vi "Main.vi"() -> ()   [LabVIEW 2021]
uses:
  Enum.ctl
  <vilib>/Instr/_visa.llb/VISA Configure Serial Port (Instr).vi
panel:
  in  "Zapisz Wykresy":bool
  in  "Wyczysc Wykresy":bool
  out "Temperatura Srednia Min [oC]":dbl
  out "PH10":cluster{"Output Value":dbl, dbl, dbl}(graph)
  out "p":cluster{"Output Value":dbl, dbl, dbl}(graph)
  out "RH":cluster{"Output Value":dbl, dbl, dbl}(graph)
  out "T":cluster{"Output Value":dbl, dbl, dbl}(graph)
  out "Iteracje Pomiarowe":i32
  out "Zapylenie Srednie Godz [ug/m3]":dbl
  out "Cisnienie Srednie Godz [hPa]":dbl
  out "Wilgotnosc Srednia Godz [%]":dbl
  out "Temperatura Srednia Godz [oC]":dbl
  out "Zapylenie Srednie Min [ug/m3]":dbl
  out "Cisnienie Srednie Min [hPa]":dbl
  out "Wilgotnosc Srednia Min [%]":dbl
  out "Zapylenie [ug/m3]":dbl
  in  "Potwierdz Haslo":bool
  in  "Haslo":string
  out "Cisnienie [hPa]":dbl
  out "Wilgotnosc [%]":dbl
  out "Temperatura [oC]":dbl
  out "Iteracje Programu":i32
  in  "Stop":bool
  in  "Arduino Port":refnum<visa-resource-name>
  # "Stacja Pogodowa"
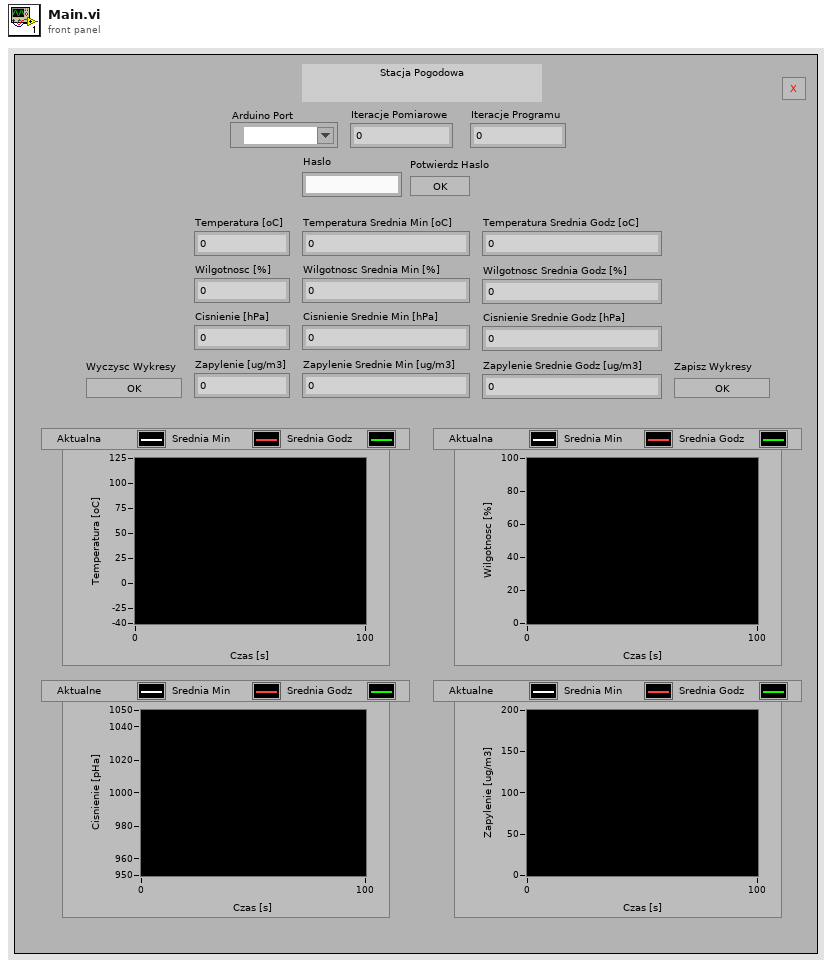
[diagram p1: front panel]
types:
  T1 = typedef "Enum.ctl" = enum16{"Init", "Password", "Measurement", "Save"}
  T2 = cluster{"Output Value":dbl, "Output Value":dbl, "Output Value":dbl, "Output Value":dbl}
  T3 = cluster{"Average 1":dbl, "Average 2":dbl, "Average 3":dbl, "Average 4":dbl}
  T4 = cluster{"Array 1":dbl[], "Array 2":dbl[], "Array 3":dbl[], "Array 4":dbl[]}
  T5 = cluster{"Output Value":dbl, "Average 1":dbl, "Average 1":dbl}
  T6 = cluster{"Output Value":dbl, "Average 2":dbl, "Average 2":dbl}
  T7 = cluster{"Output Value":dbl, "Average 3":dbl, "Average 3":dbl}
  T8 = cluster{"Output Value":dbl, "Average 4":dbl, "Average 4":dbl}
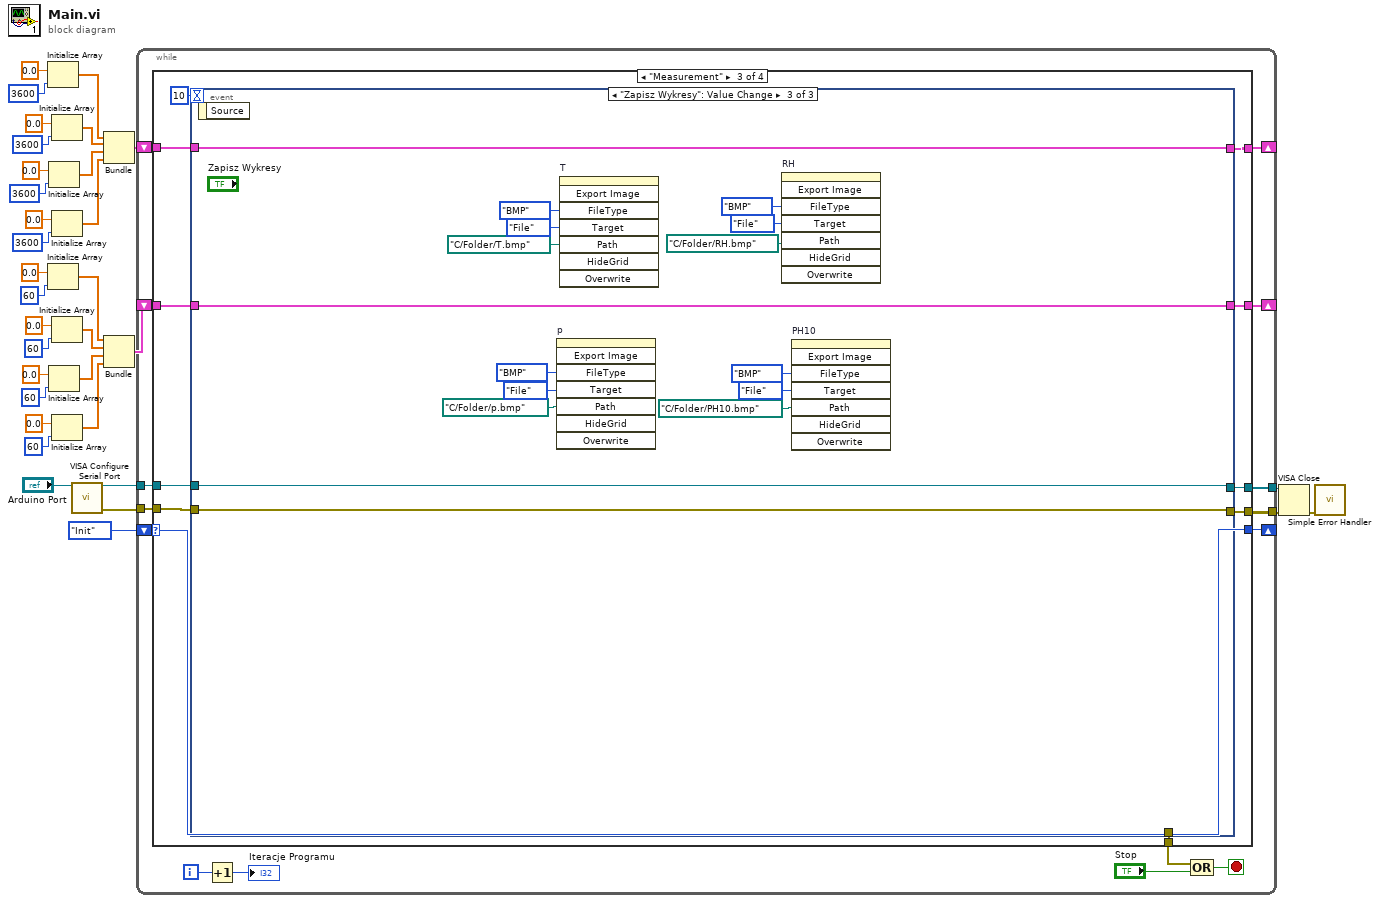
[diagram p0: block diagram]
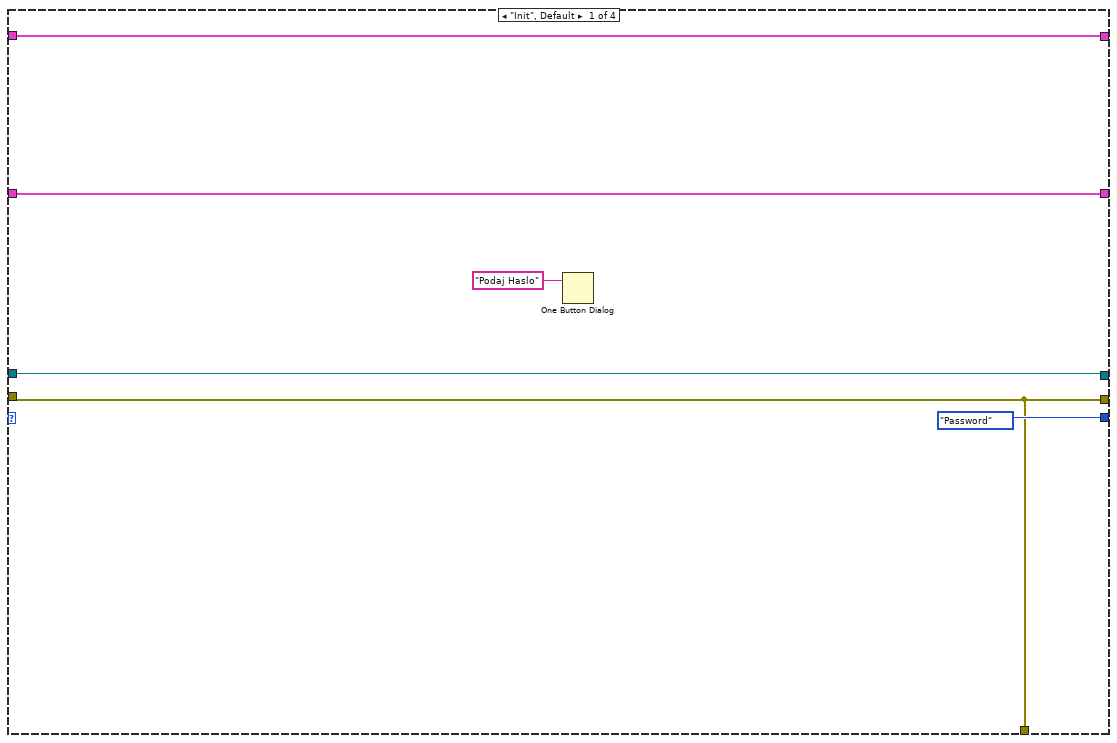
[diagram p2: hidden frame]
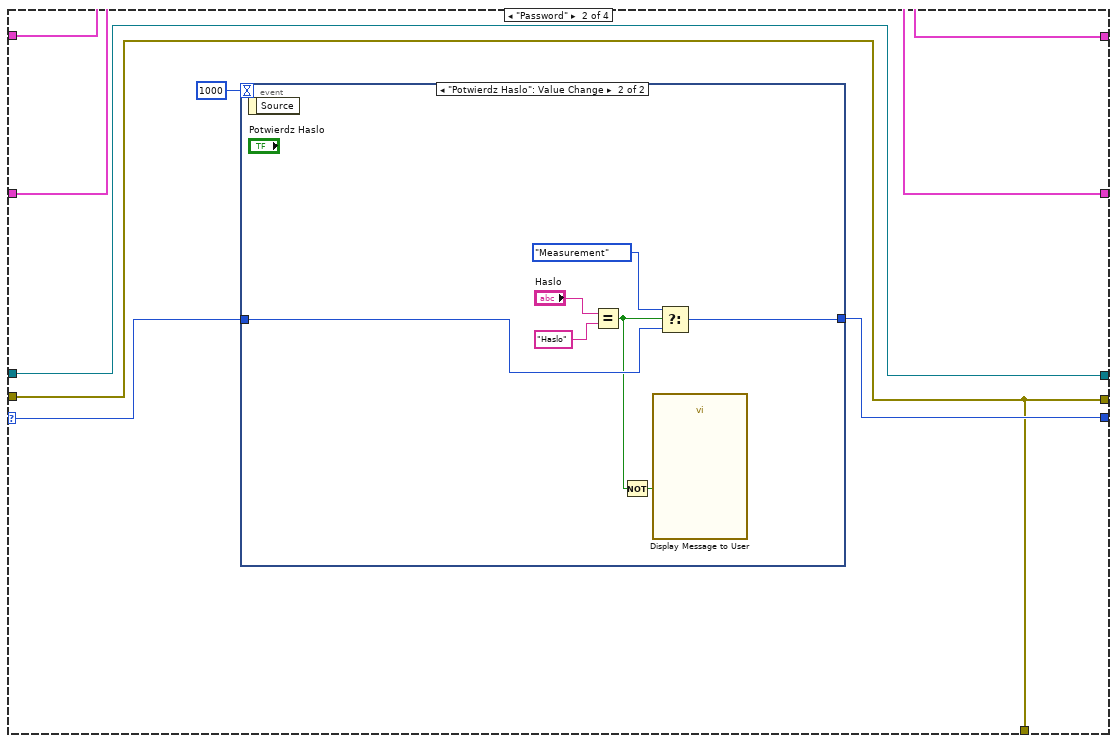
[diagram p3: hidden frame]
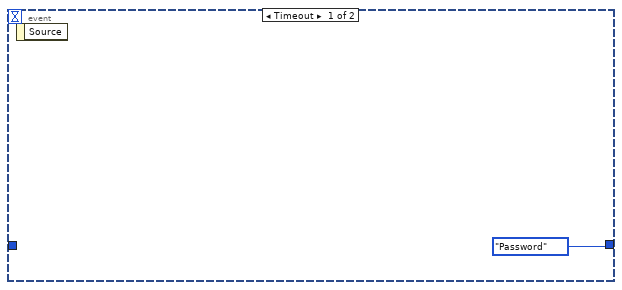
[diagram p4: hidden frame]
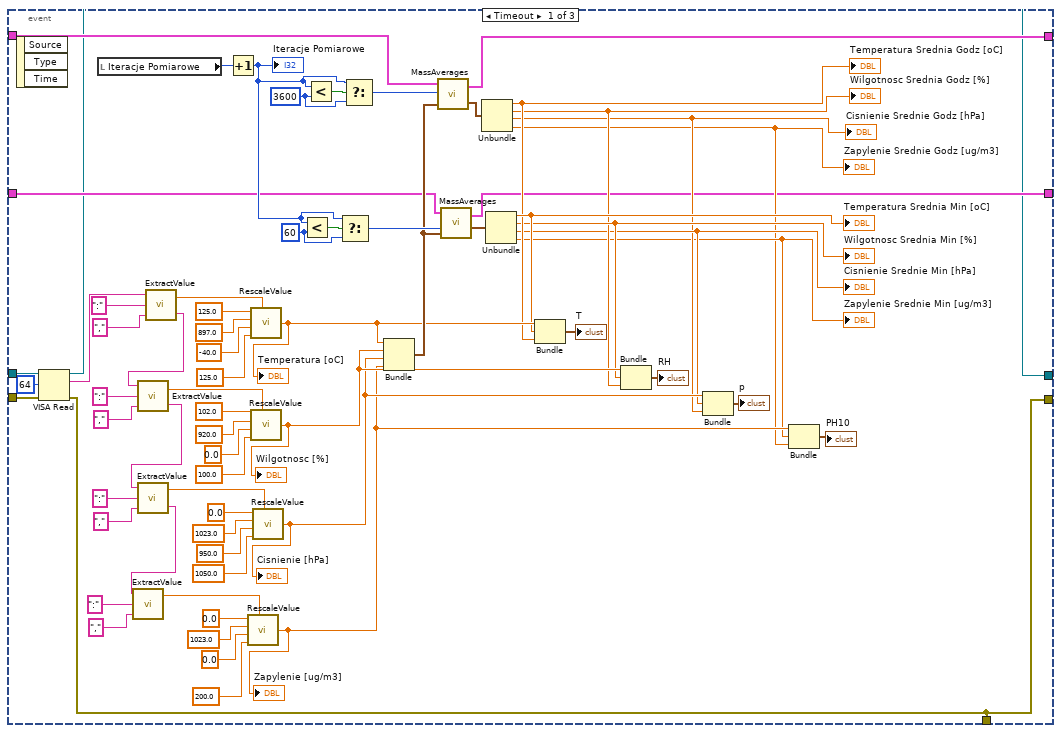
[diagram p5: hidden frame]
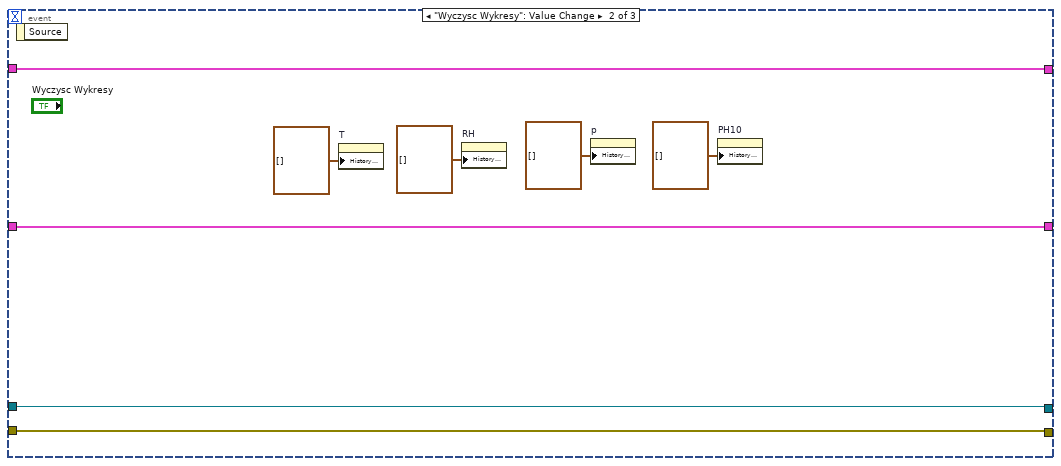
[diagram p6: hidden frame]
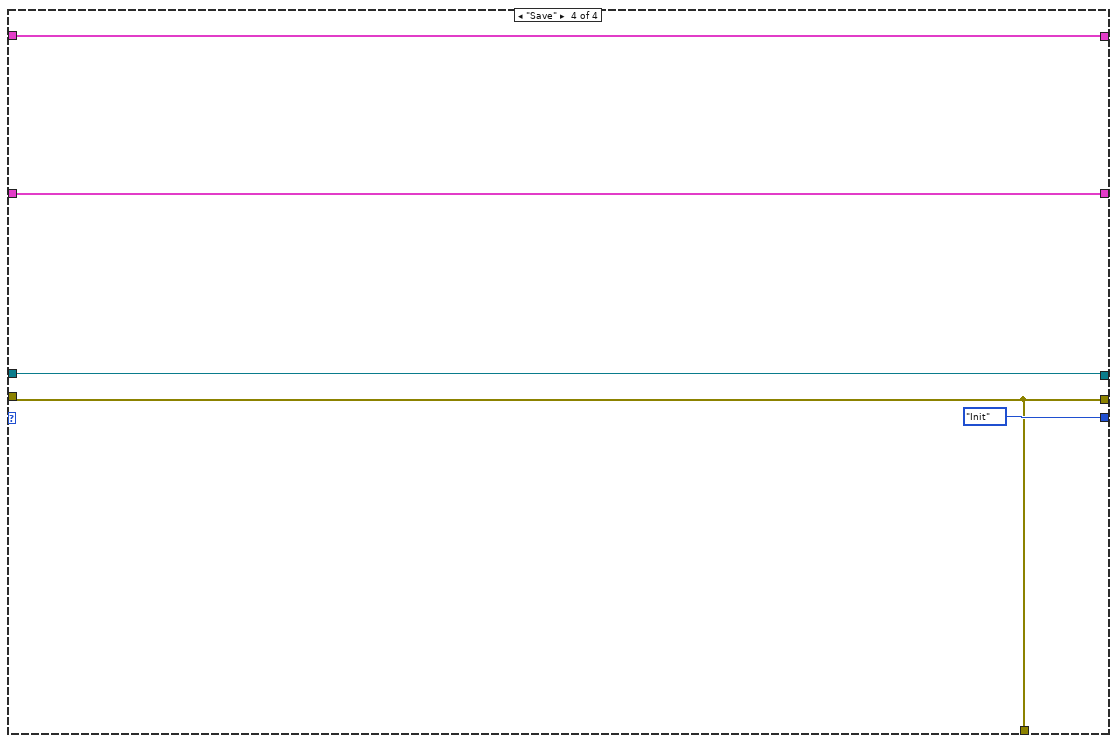
[diagram p7: hidden frame]
diagram:
  n1 = Initialize Array(0.0 ("element"), 3600 ("dimension size")) -> (w19:dbl[])
  n2 = Initialize Array(0.0 ("element"), 60 ("dimension size")) -> (w6:dbl[])
  n3 = Initialize Array(0.0 ("element"), 3600 ("dimension size")) -> (w17:dbl[])
  n4 = Initialize Array(0.0 ("element"), 60 ("dimension size")) -> (w4:dbl[])
  n5 = Initialize Array(0.0 ("element"), 3600 ("dimension size")) -> (w18:dbl[])
  n6 = Initialize Array(0.0 ("element"), 3600 ("dimension size")) -> (w16:dbl[])
  n7 = Initialize Array(0.0 ("element"), 60 ("dimension size")) -> (w5:dbl[])
  n8 = Initialize Array(0.0 ("element"), 60 ("dimension size")) -> (w3:dbl[])
  n9 = call-poly "VISA Configure Serial Port"("VISA resource name"="Arduino Port") -> ("VISA resource name out"=w33:refnum<visa-resource-name>, "error out"=w32:errorcluster)  [unwired: 13 in]
  n10 = Bundle(w19, w18, w17, w16) -> (w15:cluster{dbl[], dbl[], dbl[], dbl[]})  [unwired: 1 in]
  n11 = Bundle(w6, w5, w4, w3) -> (w2:cluster{dbl[], dbl[], dbl[], dbl[]})  [unwired: 1 in]
  n12 = while {
    tunnel: w33 -> [w43]
    tunnel: w32 -> [w41]
    shift-right: [w44] -> _
    shift-left: Enum."Init" ("Enum") -> [w45]
    tunnel: [w42] -> w29
    tunnel: [w40] -> w28
    shift-right: [w36] -> _
    shift-left: w15 -> [w37]
    shift-right: [w34] -> _
    shift-left: w2 -> [w35]
    i -> [w48]
    stop <- w47 stop-if-true
    n13 = case shown="\"Measurement\"" w45 {
      selector: w45 -> [_ w60 w80 _]
      tunnel: [Enum."Password" ("Enum") w59 w80 Enum."Init" ("Enum")] -> w44
      tunnel: w43 -> [w52 w58 w79 w176]
      tunnel: [w52 w58 w73 w176] -> w42
      tunnel: w41 -> [w51 w57 w78 w175]
      tunnel: [w51 w57 w71 w175] -> w40
      tunnel: [w51 w57 w72 w175] -> w39
      tunnel: w37 -> [w50 w56 w76 w174]
      tunnel: [w50 w56 w77 w174] -> w36
      tunnel: w35 -> [w49 w55 w75 w173]
      tunnel: [w49 w55 w74 w173] -> w34
      frame "Init", Default {
        n14 = One Button Dialog(message="Podaj Haslo") -> ()  [unwired: 1 in, 1 out]
      }
      frame "Password" {
        n15 = event shown="[1] \"Potwierdz Haslo\": Value Change" {
          selector: _ -> [_ _]
          dyn-events: _ -> [_ _]
          timeout: 1000 -> [_ _]
          tunnel: w60 -> [_ w66]
          tunnel: [Enum."Password" ("Enum") w65] -> w59
          event Timeout {
            n16 = event-data() -> ()  [unwired: 1 in, 1 out]
          }
          event "Potwierdz Haslo": Value Change {
            n17 = event-data() -> ()  [unwired: 1 in, 1 out]
            n18 = Equal?(x="Haslo", y="Haslo") -> (x = y?=w64:bool)
            n19 = Not(x=w64) -> (.not. x?=w63:bool)
            n20 = call "Display Message to User"("Enable"=w63) -> ()  [unwired: 9 in, 2 out]
            n21 = Select(t=Enum."Measurement" ("Enum"), s=w64, f=w66) -> (s? t:f=w65:T1)
          }
        }
      }
      frame "Measurement" {
        n22 = event shown="[2] \"Zapisz Wykresy\": Value Change" {
          selector: _ -> [_ _ _]
          dyn-events: _ -> [_ _ _]
          timeout: 10 -> [_ _ _]
          tunnel: w79 -> [w123 w154 w170]
          tunnel: w78 -> [w122 w153 w169]
          tunnel: [w106 w156 w172] -> w77
          tunnel: w76 -> [w105 w156 w172]
          tunnel: w75 -> [w84 w155 w171]
          tunnel: [w83 w155 w171] -> w74
          tunnel: [w82 w154 w170] -> w73
          tunnel: [w81 _ _] -> w72
          tunnel: [w81 w153 w169] -> w71
          event Timeout {
            w109 = 60 ("y")
            w111 = 3600 ("y")
            n23 = event-data() -> ()  [unwired: 1 in, 3 out]
            n24 = VISA Read(VISA resource name=w123, byte count=u32 64, error in (no error)=w122) -> (VISA resource name out=w82:refnum<visa-resource-name>, read buffer=w145:string, error out=w81:errorcluster)  [unwired: 1 out]
            n25 = local read "Iteracje Pomiarowe"() -> (w113:i32)
            n26 = call "ExtractValue.vi"("Filter 2"=",", "Filter 1"=":", "Input String"=w145) -> ("Output String"=w148:string, "Output Number"=w147:dbl)
            n27 = call "ExtractValue.vi"("Filter 2"=",", "Filter 1"=":", "Input String"=w148) -> ("Output String"=w144:string, "Output Number"=w146:dbl)
            n28 = call "ExtractValue.vi"("Filter 2"=",", "Filter 1"=":", "Input String"=w144) -> ("Output String"=w114:string, "Output Number"=w143:dbl)
            n29 = call "ExtractValue.vi"("Filter 2"=",", "Filter 1"=":", "Input String"=w114) -> ("Output Number"=w115:dbl)  [unwired: 1 out]
            n30 = Increment(x=w113) -> (x+1=w108:i32)
            "Iteracje Pomiarowe" <- w108
            n31 = call "RescaleValue.vi"("Old Scale Min"=0.0, "Old Scale Max"=1023.0, "New Scale Min"=0.0, "New Scale Max"=200.0, "Input Value"=w115) -> ("Output Value"=w88:dbl)
            "Zapylenie [ug/m3]" <- w88
            n32 = call "RescaleValue.vi"("Old Scale Min"=125.0, "Old Scale Max"=897.0, "New Scale Min"=-40.0, "New Scale Max"=125.0, "Input Value"=w147) -> ("Output Value"=w100:dbl)
            "Temperatura [oC]" <- w100
            n33 = call "RescaleValue.vi"("Old Scale Min"=102.0, "Old Scale Max"=920.0, "New Scale Min"=0.0, "New Scale Max"=100.0, "Input Value"=w146) -> ("Output Value"=w96:dbl)
            "Wilgotnosc [%]" <- w96
            n34 = call "RescaleValue.vi"("Old Scale Min"=0.0, "Old Scale Max"=1023.0, "New Scale Min"=950.0, "New Scale Max"=1050.0, "Input Value"=w143) -> ("Output Value"=w92:dbl)
            "Cisnienie [hPa]" <- w92
            n35 = Less?(x=w108, y=w109) -> (x < y?=w110:bool)
            n36 = Less?(x=w108, y=w111) -> (x < y?=w112:bool)
            n37 = Select(t=w108, s=w110, f=w109) -> (s? t:f=w104:i32)
            n38 = Select(t=w108, s=w112, f=w111) -> (s? t:f=w107:i32)
            n39 = Bundle("Output Value"=w100, "Output Value"=w96, "Output Value"=w92, "Output Value"=w88) -> (w101:T2)  [unwired: 1 in]
            n40 = call "MassAverages.vi"("Input Cluster"=w101, "N"=w107, "Array In Cluster"=w105) -> ("Average Cluster"=w102:T3, "Array Out Cluster"=w106:T4)
            n41 = call "MassAverages.vi"("Input Cluster"=w101, "N"=w104, "Array In Cluster"=w84) -> ("Average Cluster"=w103:T3, "Array Out Cluster"=w83:T4)
            n42 = Unbundle(w102) -> ("Average 1"=w98:dbl, "Average 2"=w94:dbl, "Average 3"=w90:dbl, "Average 4"=w86:dbl)
            "Temperatura Srednia Godz [oC]" <- w98
            "Wilgotnosc Srednia Godz [%]" <- w94
            "Cisnienie Srednie Godz [hPa]" <- w90
            "Zapylenie Srednie Godz [ug/m3]" <- w86
            n43 = Unbundle(w103) -> ("Average 1"=w99:dbl, "Average 2"=w95:dbl, "Average 3"=w91:dbl, "Average 4"=w87:dbl)
            "Wilgotnosc Srednia Min [%]" <- w95
            "Cisnienie Srednie Min [hPa]" <- w91
            "Zapylenie Srednie Min [ug/m3]" <- w87
            "Temperatura Srednia Min [oC]" <- w99
            n44 = Bundle("Output Value"=w100, "Average 1"=w99, "Average 1"=w98) -> (→"T":T5)  [unwired: 1 in]
            n45 = Bundle("Output Value"=w96, "Average 2"=w95, "Average 2"=w94) -> (→"RH":T6)  [unwired: 1 in]
            n46 = Bundle("Output Value"=w92, "Average 3"=w91, "Average 3"=w90) -> (→"p":T7)  [unwired: 1 in]
            n47 = Bundle("Output Value"=w88, "Average 4"=w87, "Average 4"=w86) -> (→"PH10":T8)  [unwired: 1 in]
          }
          event "Wyczysc Wykresy": Value Change {
            n48 = event-data() -> ()  [unwired: 1 in, 1 out]
            n49 = property on="T" class="WFChart (strict)"("History Data"=cluster{"Output Value":dbl, dbl, dbl}[] []) -> ()  [unwired: 2 in, 2 out]
            n50 = property on="RH" class="WFChart (strict)"("History Data"=cluster{"Output Value":dbl, dbl, dbl}[] []) -> ()  [unwired: 2 in, 2 out]
            n51 = property on="p" class="WFChart (strict)"("History Data"=cluster{"Output Value":dbl, dbl, dbl}[] []) -> ()  [unwired: 2 in, 2 out]
            n52 = property on="PH10" class="WFChart (strict)"("History Data"=cluster{"Output Value":dbl, dbl, dbl}[] []) -> ()  [unwired: 2 in, 2 out]
          }
          event "Zapisz Wykresy": Value Change {
            n53 = event-data() -> ()  [unwired: 1 in, 1 out]
            n54 = invoke on="p" class="WFChart (strict)" method="Export Image"("FileType"=enum32{"BMP", "EPS", "EMF", "PICT"}."BMP" ("File Type"), "Target"=enum32{"File", "Clipboard"}."File", "Path"=path "C:/Folder/p.bmp") -> ()  [unwired: 5 in, 8 out]
            n55 = invoke on="T" class="WFChart (strict)" method="Export Image"("FileType"=enum32{"BMP", "EPS", "EMF", "PICT"}."BMP" ("File Type"), "Target"=enum32{"File", "Clipboard"}."File", "Path"=path "C:/Folder/T.bmp") -> ()  [unwired: 5 in, 8 out]
            n56 = invoke on="RH" class="WFChart (strict)" method="Export Image"("FileType"=enum32{"BMP", "EPS", "EMF", "PICT"}."BMP" ("File Type"), "Target"=enum32{"File", "Clipboard"}."File", "Path"=path "C:/Folder/RH.bmp") -> ()  [unwired: 5 in, 8 out]
            n57 = invoke on="PH10" class="WFChart (strict)" method="Export Image"("FileType"=enum32{"BMP", "EPS", "EMF", "PICT"}."BMP" ("File Type"), "Target"=enum32{"File", "Clipboard"}."File", "Path"=path "C:/Folder/PH10.bmp") -> ()  [unwired: 5 in, 8 out]
          }
        }
      }
      frame "Save" {
      }
    }
    n58 = Increment(x=w48) -> (x+1=→"Iteracje Programu":i32)
    n59 = Compound Arithmetic op=OR(w39, "Stop") -> (w47:bool)
  }
  n60 = VISA Close(VISA resource name=w29, error in (no error)=w28) -> (error out=w1:errorcluster)
  n61 = call <vilib>:"Simple Error Handler.vi"("error in (no error)"=w1) -> ()  [unwired: 4 in, 5 out]
